vi "SetValueForListBox.vi"(0 "Control Ref In":refnum<vi>, 5 "Value (Signaling)":variant, 11 "Error In":errorcluster) -> (4 "Control Ref Out":refnum<vi>, 15 "Error Out":errorcluster)   [LabVIEW 2016, in "Drona.lvlib" / "ControlValue.lvlib"]
doc: "Sets the specified value on listbox control"
uses:
  ControlValue.lvlib
  <vilib>/Utility/error.llb/Error Cluster From Error Code.vi
  <vilib>/ErrorRing/Error Ring.xnode
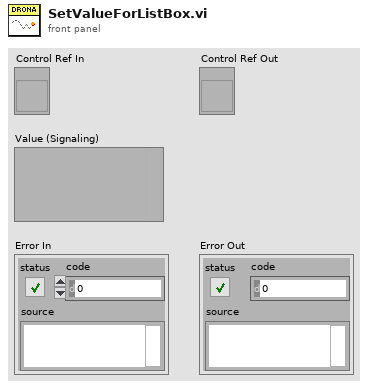
[diagram p1: front panel]
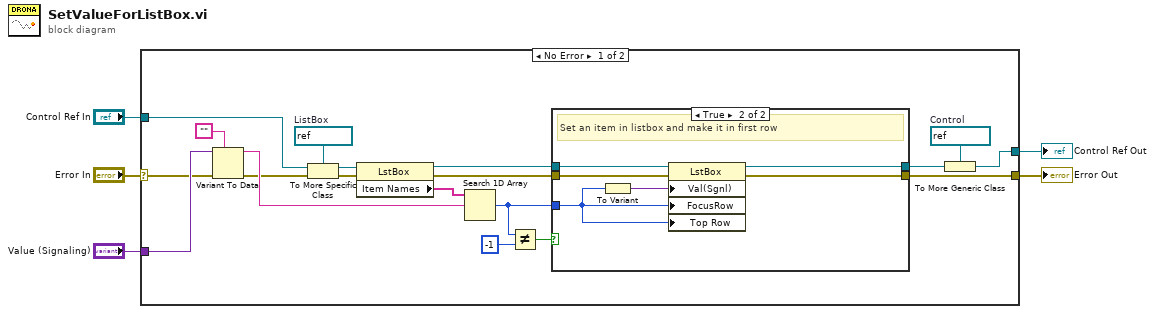
[diagram p0: block diagram]
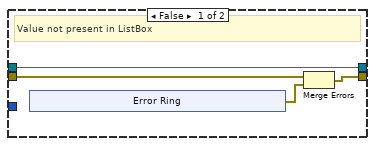
[diagram p2: hidden frame]
diagram:
  n1 = case shown="No Error" "Error In" {
    selector: "Error In" -> [w9 w40]
    tunnel: [w24 w41] -> w5
    tunnel: [w20 w40] -> w4
    tunnel: "Control Ref In" -> [w19 w41]
    tunnel: "Value (Signaling)" -> [w16 _]
    frame No Error {
      w23 = refnum<vi> refnum  # Control
      w11 = refnum<vi> refnum  # ListBox
      n2 = To More Specific Class(target class=w11, reference=w19, error in=w9) -> (specific class reference=w13:refnum<vi>, error out=w10:errorcluster)
      n3 = property class="LstBox"(reference=w13, error in=w10) -> (reference out=w21:refnum<vi>, error out=w12:errorcluster, "Item Names"=w14:string[])
      n4 = Variant To Data(error in=w12, type="", Variant=w16) -> (data=w18:string, error out=w15:errorcluster)
      n5 = Search 1D Array(1D array=w14, element=w18) -> (index of element=w8:i32)  [unwired: 1 in]
      n6 = Not Equal?(x=w8, y=-1) -> (x != y?=w6:bool)
      n7 = case shown="True" w6 {
        tunnel: [w28 w39] -> w22
        tunnel: w21 -> [w28 w37]
        tunnel: [w26 w36] -> w20
        tunnel: w15 -> [w27 w35]
        tunnel: w8 -> [_ w34]
        frame False {
          # "Value not present in ListBox"
          n8 = xnode "Error Ring"() -> ("error out"=w25:errorcluster)
          n9 = Merge Errors(w27, w25) -> (w26:errorcluster)
        }
        frame True {
          # "Set an item in listbox and make it in first row"
          n10 = To Variant(anything=w34) -> (Variant=w38:variant)
          n11 = property class="LstBox"(reference=w37, error in=w35, "Val(Sgnl)"=w38, "FocusRow"=w34, "Top Row"=w34) -> (reference out=w39:refnum<vi>, error out=w36:errorcluster)
        }
      }
      n12 = To More Generic Class(target class=w23, reference=w22) -> (generic class reference=w24:refnum<vi>)
    }
    frame Error {
    }
  }
  "Control Ref Out" <- w5
  "Error Out" <- w4
